vi "Destroy.vi"(8 "error in":errorcluster, 11 "message ref in":refnum<class "CLM_LocalMessage.lvclass">) -> (0 "error out":errorcluster)   [LabVIEW 2013, in "CLM_LocalMessage.lvclass"]
uses:
  CLM_LocalMessage.lvclass
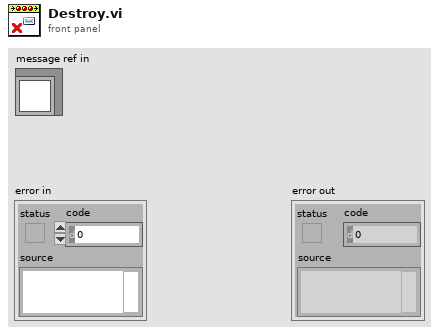
[diagram p1: front panel]
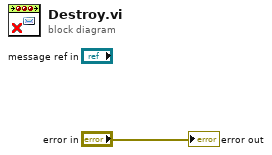
[diagram p0: block diagram]
diagram:
  "error out" <- "error in"
